vi "BotSpeak_FILE READ.vi"(2 "file name":string="test.htm", 4 "Bot Settings":T1) -> (0 "response":string="Test", 1 "Bot Settings 2":T1)   [LabVIEW 2014]
doc: "Reads the html associated with the RIO, returned as \"response\"."
uses:
  <userlib>/botspeak/VIs/Direct/BotSpeak_Control.ctl
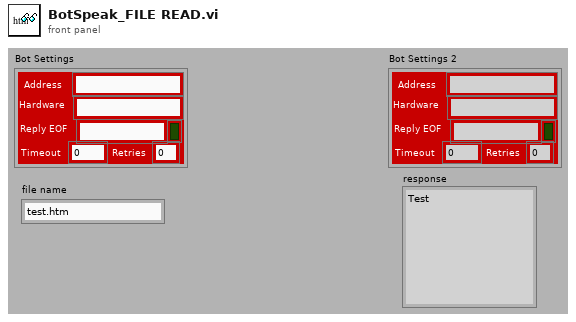
[diagram p1: front panel]
types:
  T1 = typedef "BotSpeak_Control.ctl" = cluster{"Address":string, "Reply EOF":string, "Hardware":string, "Retries":i8, "Timeout":i32, "Open?":bool}
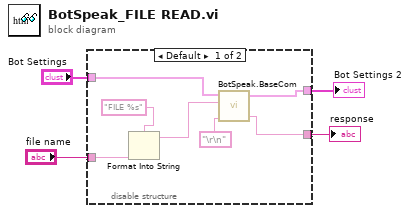
[diagram p0: block diagram]
diagram:
  n1 = disable-structure shown="Default" {
    disable-tunnel: "file name" -> [w11 _]
    disable-tunnel: "Bot Settings" -> [w9 _]
    disable-tunnel: [w8 _] -> w2
    disable-tunnel: [w6 _] -> w1
    frame condition #0 {
      n2 = Format Into String(format string="FILE %s" ("command"), w11) -> (resulting string=w7:string)  [unwired: 2 in, 1 out]
      n3 = call <userlib>:"BotSpeak.BaseCom.vi"("Termination"="\r\n", "command"=w7, "Bot Settings in"=w9) -> ("response"=w6:string, "Bot Settings out"=w8:T1)  [unwired: 2 in]
    }
    frame condition #1 (active) {
    }
  }
  "response" <- w1
  "Bot Settings 2" <- w2
